vi "JSON to LVObject.vi"(7 "Class 1 in":refnum<class "Serializer-Scheme.lvclass">, 8 "error in":errorcluster, 9 "Object Type":refnum<class>, 10 "Offset":i32, 11 "JSON":string) -> (0 "error out":errorcluster, 1 "Object":refnum<class>)   [LabVIEW 2021, in "TSC Material Theme.lvlib" / "Serializer-Scheme.lvclass"]
doc: "Convert JSON to an Object of a LabVIEW Class."
uses:
  Serializer-Scheme.lvclass
  TSC Material Theme/material json scheme--cluster.ctl
  Material-Scheme/Material-Scheme.lvclass
  Serializer-Scheme.lvclass/Serializer-Scheme.ctl
  Material-Scheme/Material-Scheme.lvclass/Material-Scheme.ctl
  Material-Scheme/data member access/Set name.vi
  Material-Scheme/data member access/Set primary.vi
  Material-Scheme/data member access/Set surfaceTint.vi
  Material-Scheme/data member access/Set onPrimary.vi
  Material-Scheme/data member access/Set primaryContainer.vi
  Material-Scheme/data member access/Set onPrimaryContainer.vi
  Material-Scheme/data member access/Set secondary.vi
  Material-Scheme/data member access/Set onSecondary.vi
  Material-Scheme/data member access/Set secondaryContainer.vi
  Material-Scheme/data member access/Set onSecondaryContainer.vi
  Material-Scheme/data member access/Set tertiary.vi
  Material-Scheme/data member access/Set onTertiary.vi
  Material-Scheme/data member access/Set tertiaryContainer.vi
  Material-Scheme/data member access/Set onTertiaryContainer.vi
  Material-Scheme/data member access/Set error.vi
  Material-Scheme/data member access/Set onError.vi
  Material-Scheme/data member access/Set errorContainer.vi
  Material-Scheme/data member access/Set onErrorContainer.vi
  Material-Scheme/data member access/Set background.vi
  Material-Scheme/data member access/Set onBackground.vi
  Material-Scheme/data member access/Set surface.vi
  Material-Scheme/data member access/Set onSurface.vi
  Material-Scheme/data member access/Set surfaceVariant.vi
  Material-Scheme/data member access/Set onSurfaceVariant.vi
  Material-Scheme/data member access/Set outline.vi
  Material-Scheme/data member access/Set outlineVariant.vi
  Material-Scheme/data member access/Set shadow.vi
  Material-Scheme/data member access/Set scrim.vi
  Material-Scheme/data member access/Set inverseSurface.vi
  Material-Scheme/data member access/Set inverseOnSurface.vi
  Material-Scheme/data member access/Set inversePrimary.vi
  Material-Scheme/data member access/Set primaryFixed.vi
  Material-Scheme/data member access/Set onPrimaryFixed.vi
  Material-Scheme/data member access/Set primaryFixedDim.vi
  Material-Scheme/data member access/Set onPrimaryFixedVariant.vi
  Material-Scheme/data member access/Set secondaryFixed.vi
  Material-Scheme/data member access/Set onSecondaryFixed.vi
  Material-Scheme/data member access/Set secondaryFixedDim.vi
  Material-Scheme/data member access/Set onSecondaryFixedVariant.vi
  Material-Scheme/data member access/Set tertiaryFixed.vi
  Material-Scheme/data member access/Set onTertiaryFixed.vi
  Material-Scheme/data member access/Set tertiaryFixedDim.vi
  Material-Scheme/data member access/Set onTertiaryFixedVariant.vi
  Material-Scheme/data member access/Set surfaceDim.vi
  Material-Scheme/data member access/Set surfaceBright.vi
  Material-Scheme/data member access/Set surfaceContainerLowest.vi
  Material-Scheme/data member access/Set surfaceContainerLow.vi
  Material-Scheme/data member access/Set surfaceContainer.vi
  Material-Scheme/data member access/Set surfaceContainerHigh.vi
  Material-Scheme/data member access/Set surfaceContainerHighest.vi
  <vilib>/JDP Science/JSONtext/JSONtext.lvlib
  TSC Material Theme/TSC Material Theme.lvlib
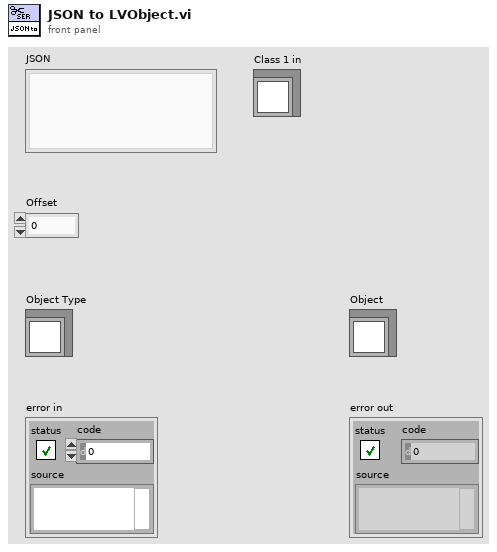
[diagram p1: front panel]
types:
  T1 = typedef "TSC Material Theme.lvlib/material json scheme--cluster.ctl" = cluster{"primary":string, "surfaceTint":string, "onPrimary":string, "primaryContainer":string, "onPrimaryContainer":string, "secondary":string, "onSecondary":string, "secondaryContainer":string, "onSecondaryContainer":string, "tertiary":string, "onTertiary":string, "tertiaryContainer":string, "onTertiaryContainer":string, "error":string, "onError":string, "errorContainer":string, "onErrorContainer":string, "background":string, "onBackground":string, "surface":string, "onSurface":string, "surfaceVariant":string, "onSurfaceVariant":string, "outline":string, "outlineVariant":string, "shadow":string, "scrim":string, "inverseSurface":string, "inverseOnSurface":string, "inversePrimary":string, "primaryFixed":string, "onPrimaryFixed":string, "primaryFixedDim":string, "onPrimaryFixedVariant":string, "secondaryFixed":string, "onSecondaryFixed":string, "secondaryFixedDim":string, "onSecondaryFixedVariant":string, "tertiaryFixed":string, "onTertiaryFixed":string, "tertiaryFixedDim":string, "onTertiaryFixedVariant":string, "surfaceDim":string, "surfaceBright":string, "surfaceContainerLowest":string, "surfaceContainerLow":string, "surfaceContainer":string, "surfaceContainerHigh":string, "surfaceContainerHighest":string}
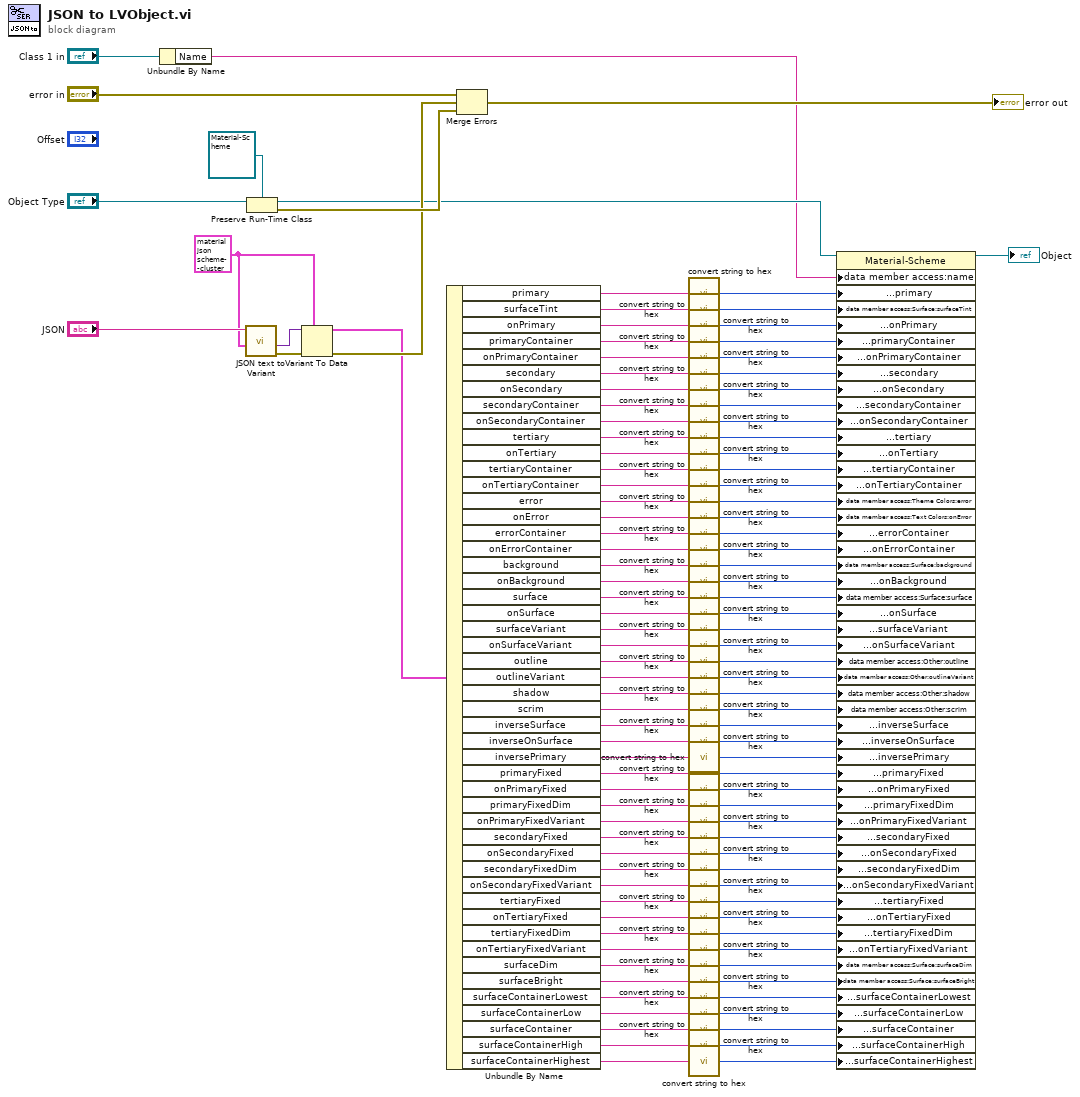
[diagram p0: block diagram]
diagram:
  w104 = T1 {"primary"="", "surfaceTint"="", "onPrimary"="", "primaryContainer"="", "onPrimaryContainer"="", "secondary"="", "onSecondary"="", "secondaryContainer"="", "onSecondaryContainer"="", "tertiary"="", "onTertiary"="", "tertiaryContainer"="", "onTertiaryContainer"="", "error"="", "onError"="", "errorContainer"="", "onErrorContainer"="", "background"="", "onBackground"="", "surface"="", "onSurface"="", "surfaceVariant"="", "onSurfaceVariant"="", "outline"="", "outlineVariant"="", "shadow"="", "scrim"="", "inverseSurface"="", "inverseOnSurface"="", "inversePrimary"="", "primaryFixed"="", "onPrimaryFixed"="", "primaryFixedDim"="", "onPrimaryFixedVariant"="", "secondaryFixed"="", "onSecondaryFixed"="", "secondaryFixedDim"="", "onSecondaryFixedVariant"="", "tertiaryFixed"="", "onTertiaryFixed"="", "tertiaryFixedDim"="", "onTertiaryFixedVariant"="", "surfaceDim"="", "surfaceBright"="", "surfaceContainerLowest"="", "surfaceContainerLow"="", "surfaceContainer"="", "surfaceContainerHigh"="", "surfaceContainerHighest"=""} ("light")
  n1 = Unbundle By Name("Class 1 in") -> ("Name"=w1:string)
  n2 = call <vilib>:"JSON text to Variant.vi"("Data Type"=w104, "JSON"="JSON") -> ("error out"=w113:errorcluster, "Variant out"=w105:variant)  [unwired: 8 in]
  n3 = Preserve Run-Time Class(object in="Object Type", 2:refnum<class "Material-Scheme.lvclass"> refnum ("TSC Material Theme.lvlib:Material-Scheme")) -> (object out=w49:refnum<class "Material-Scheme.lvclass">, error out=w111:errorcluster)  [unwired: 1 in]
  n4 = Variant To Data(error in=w113, type=w104, Variant=w105) -> (data=w55:T1, error out=w110:errorcluster)
  n5 = Unbundle By Name(w55) -> ("primary"=w54:string, "surfaceTint"=w103:string, "onPrimary"=w102:string, "primaryContainer"=w101:string, "onPrimaryContainer"=w100:string, "secondary"=w99:string, "onSecondary"=w98:string, "secondaryContainer"=w97:string, "onSecondaryContainer"=w96:string, "tertiary"=w95:string, "onTertiary"=w94:string, "tertiaryContainer"=w93:string, "onTertiaryContainer"=w92:string, "error"=w91:string, "onError"=w90:string, "errorContainer"=w89:string, "onErrorContainer"=w88:string, "background"=w87:string, "onBackground"=w86:string, "surface"=w85:string, "onSurface"=w84:string, "surfaceVariant"=w83:string, "onSurfaceVariant"=w82:string, "outline"=w81:string, "outlineVariant"=w80:string, "shadow"=w79:string, "scrim"=w78:string, "inverseSurface"=w77:string, "inverseOnSurface"=w76:string, "inversePrimary"=w56:string, "primaryFixed"=w75:string, "onPrimaryFixed"=w74:string, "primaryFixedDim"=w73:string, "onPrimaryFixedVariant"=w72:string, "secondaryFixed"=w71:string, "onSecondaryFixed"=w70:string, "secondaryFixedDim"=w69:string, "onSecondaryFixedVariant"=w68:string, "tertiaryFixed"=w67:string, "onTertiaryFixed"=w66:string, "tertiaryFixedDim"=w65:string, "onTertiaryFixedVariant"=w64:string, "surfaceDim"=w63:string, "surfaceBright"=w62:string, "surfaceContainerLowest"=w61:string, "surfaceContainerLow"=w60:string, "surfaceContainer"=w59:string, "surfaceContainerHigh"=w58:string, "surfaceContainerHighest"=w57:string)
  n6 = Merge Errors("error in", w110, w111) -> (→"error out":errorcluster)
  n7 = call "convert string to hex.vi"("string"=w54) -> ("hex"=w53:u32)
  n8 = call "convert string to hex.vi"("string"=w103) -> ("hex"=w52:u32)
  n9 = call "convert string to hex.vi"("string"=w102) -> ("hex"=w51:u32)
  n10 = call "convert string to hex.vi"("string"=w101) -> ("hex"=w48:u32)
  n11 = call "convert string to hex.vi"("string"=w100) -> ("hex"=w47:u32)
  n12 = call "convert string to hex.vi"("string"=w99) -> ("hex"=w46:u32)
  n13 = call "convert string to hex.vi"("string"=w98) -> ("hex"=w45:u32)
  n14 = call "convert string to hex.vi"("string"=w97) -> ("hex"=w44:u32)
  n15 = call "convert string to hex.vi"("string"=w96) -> ("hex"=w43:u32)
  n16 = call "convert string to hex.vi"("string"=w95) -> ("hex"=w42:u32)
  n17 = call "convert string to hex.vi"("string"=w94) -> ("hex"=w41:u32)
  n18 = call "convert string to hex.vi"("string"=w93) -> ("hex"=w40:u32)
  n19 = call "convert string to hex.vi"("string"=w92) -> ("hex"=w39:u32)
  n20 = call "convert string to hex.vi"("string"=w91) -> ("hex"=w38:u32)
  n21 = call "convert string to hex.vi"("string"=w90) -> ("hex"=w37:u32)
  n22 = call "convert string to hex.vi"("string"=w89) -> ("hex"=w36:u32)
  n23 = call "convert string to hex.vi"("string"=w88) -> ("hex"=w35:u32)
  n24 = call "convert string to hex.vi"("string"=w87) -> ("hex"=w34:u32)
  n25 = call "convert string to hex.vi"("string"=w86) -> ("hex"=w33:u32)
  n26 = call "convert string to hex.vi"("string"=w85) -> ("hex"=w32:u32)
  n27 = call "convert string to hex.vi"("string"=w84) -> ("hex"=w31:u32)
  n28 = call "convert string to hex.vi"("string"=w83) -> ("hex"=w30:u32)
  n29 = call "convert string to hex.vi"("string"=w82) -> ("hex"=w29:u32)
  n30 = call "convert string to hex.vi"("string"=w81) -> ("hex"=w28:u32)
  n31 = call "convert string to hex.vi"("string"=w80) -> ("hex"=w27:u32)
  n32 = call "convert string to hex.vi"("string"=w79) -> ("hex"=w26:u32)
  n33 = call "convert string to hex.vi"("string"=w78) -> ("hex"=w25:u32)
  n34 = call "convert string to hex.vi"("string"=w77) -> ("hex"=w24:u32)
  n35 = call "convert string to hex.vi"("string"=w76) -> ("hex"=w23:u32)
  n36 = call "convert string to hex.vi"("string"=w56) -> ("hex"=w22:u32)
  n37 = call "convert string to hex.vi"("string"=w75) -> ("hex"=w21:u32)
  n38 = call "convert string to hex.vi"("string"=w74) -> ("hex"=w20:u32)
  n39 = call "convert string to hex.vi"("string"=w73) -> ("hex"=w19:u32)
  n40 = call "convert string to hex.vi"("string"=w72) -> ("hex"=w18:u32)
  n41 = call "convert string to hex.vi"("string"=w71) -> ("hex"=w17:u32)
  n42 = call "convert string to hex.vi"("string"=w70) -> ("hex"=w16:u32)
  n43 = call "convert string to hex.vi"("string"=w69) -> ("hex"=w15:u32)
  n44 = call "convert string to hex.vi"("string"=w68) -> ("hex"=w14:u32)
  n45 = call "convert string to hex.vi"("string"=w67) -> ("hex"=w3:u32)
  n46 = call "convert string to hex.vi"("string"=w66) -> ("hex"=w4:u32)
  n47 = call "convert string to hex.vi"("string"=w65) -> ("hex"=w5:u32)
  n48 = call "convert string to hex.vi"("string"=w64) -> ("hex"=w6:u32)
  n49 = call "convert string to hex.vi"("string"=w63) -> ("hex"=w7:u32)
  n50 = call "convert string to hex.vi"("string"=w62) -> ("hex"=w8:u32)
  n51 = call "convert string to hex.vi"("string"=w61) -> ("hex"=w9:u32)
  n52 = call "convert string to hex.vi"("string"=w60) -> ("hex"=w10:u32)
  n53 = call "convert string to hex.vi"("string"=w59) -> ("hex"=w11:u32)
  n54 = call "convert string to hex.vi"("string"=w58) -> ("hex"=w12:u32)
  n55 = call "convert string to hex.vi"("string"=w57) -> ("hex"=w13:u32)
  n56 = property class="Material-Scheme"(reference=w49, "data member access:name"=w1, "data member access:Theme Colors:primary"=w53, "data member access:Surface:surfaceTint"=w52, "data member access:Text Colors:onPrimary"=w51, "data member access:Theme Colors:primaryContainer"=w48, "data member access:Text Colors:onPrimaryContainer"=w47, "data member access:Theme Colors:secondary"=w46, "data member access:Text Colors:onSecondary"=w45, "data member access:Theme Colors:secondaryContainer"=w44, "data member access:Text Colors:onSecondaryContainer"=w43, "data member access:Theme Colors:tertiary"=w42, "data member access:Text Colors:onTertiary"=w41, "data member access:Theme Colors:tertiaryContainer"=w40, "data member access:Text Colors:onTertiaryContainer"=w39, "data member access:Theme Colors:error"=w38, "data member access:Text Colors:onError"=w37, "data member access:Theme Colors:errorContainer"=w36, "data member access:Text Colors:onErrorContainer"=w35, "data member access:Surface:background"=w34, "data member access:Text Colors:onBackground"=w33, "data member access:Surface:surface"=w32, "data member access:Text Colors:onSurface"=w31, "data member access:Surface:surfaceVariant"=w30, "data member access:Text Colors:onSurfaceVariant"=w29, "data member access:Other:outline"=w28, "data member access:Other:outlineVariant"=w27, "data member access:Other:shadow"=w26, "data member access:Other:scrim"=w25, "data member access:Surface:inverseSurface"=w24, "data member access:Text Colors:inverseOnSurface"=w23, "data member access:Theme Colors:inversePrimary"=w22, "data member access:Fixed Colors:primaryFixed"=w21, "data member access:Text Colors Fixed:onPrimaryFixed"=w20, "data member access:Fixed Colors:primaryFixedDim"=w19, "data member access:Text Colors Fixed:onPrimaryFixedVariant"=w18, "data member access:Fixed Colors:secondaryFixed"=w17, "data member access:Text Colors Fixed:onSecondaryFixed"=w16, "data member access:Fixed Colors:secondaryFixedDim"=w15, "data member access:Text Colors Fixed:onSecondaryFixedVariant"=w14, "data member access:Fixed Colors:tertiaryFixed"=w3, "data member access:Text Colors Fixed:onTertiaryFixed"=w4, "data member access:Fixed Colors:tertiaryFixedDim"=w5, "data member access:Text Colors Fixed:onTertiaryFixedVariant"=w6, "data member access:Surface:surfaceDim"=w7, "data member access:Surface:surfaceBright"=w8, "data member access:Surface:surfaceContainerLowest"=w9, "data member access:Surface:surfaceContainerLow"=w10, "data member access:Surface:surfaceContainer"=w11, "data member access:Surface:surfaceContainerHigh"=w12, "data member access:Surface:surfaceContainerHighest"=w13) -> (reference out=→"Object":refnum<class "Material-Scheme.lvclass">)  [unwired: 1 in, 1 out]
